vi "Get Index.vi"(8 "Error In":errorcluster, 11 "reference in":refnum<class "OD Entry.lvclass">) -> (0 "Error Out":errorcluster, 2 "Index":u16 format="%.0x", 3 "reference out":refnum<class "OD Entry.lvclass">)   [LabVIEW 2024, in "Electronic Datasheet.lvlib" / "OD Entry.lvclass"]
uses:
  OD Entry.lvclass
  OD Entry.lvclass/OD Entry.ctl
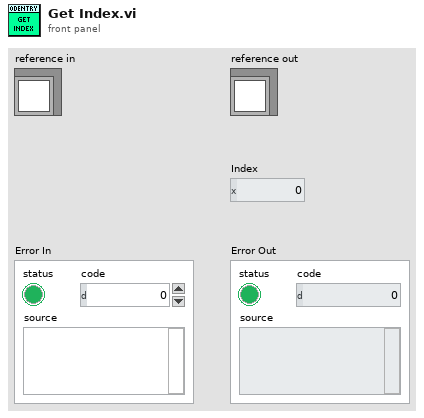
[diagram p1: front panel]
types:
  T1 = typedef "Electronic Datasheet.lvlib/OD Entry.lvclass/ObjectAttributes.ctl" = cluster{"Index":u16, "ObjectType":refnum<class "Object Type Base.lvclass">, "Denotation":string, "Count":u8, "ObjExtend":u8, "PDOtype":T2, "Label":string, "Description":string, "Sub-Entries":map{u8, refnum<class "OD Sub-Entry.lvclass">}}
  T2 = typedef "Electronic Datasheet.lvlib/PDO Mapping Type.ctl" = enum16{"NO", "OPTIONAL", "RPDO", "TPDO", "DEFAULT"}
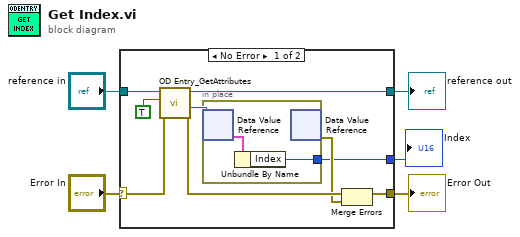
[diagram p0: block diagram]
diagram:
  n1 = case shown="No Error" "Error In" {
    selector: "Error In" -> [w14 w18]
    tunnel: [w12 w18] -> w4
    tunnel: [w9 w17] -> w2
    tunnel: "reference in" -> [w10 w17]
    tunnel: [w6 _] -> w1
    frame No Error {
      n2 = call "OD Entry_GetAttributes.vi"("Error In"=w14, "OnlyGetDvrReference(False)"=TRUE, "reference in"=w10) -> ("Error Out"=w13:errorcluster, "DataRef"=w7:refnum<data-value>, "reference out"=w9:refnum<class "OD Entry.lvclass">)  [unwired: 5 in, 1 out]
      n3 = in-place {
        in-place-border: [w16] -> w6
        n4 = in-place-dvr #1(w7) -> (w15:T1)  [unwired: 1 out]
        n5 = Unbundle By Name(w15) -> ("Index"=w16:u16)
        n6 = in-place-dvr #1() -> (w11:errorcluster)  [unwired: 1 in, 1 out]
      }
      n7 = Merge Errors(w13, w11) -> (w12:errorcluster)
    }
    frame Error {
    }
  }
  "Error Out" <- w4
  "reference out" <- w2
  "Index" <- w1
